vi "UpdateErrorfile.vi"(8 "error in (no error)":errorcluster, 9 "Error file number":u32, 10 "Error file":path, 11 "TCP_serverGUI in":refnum<class "TCP_serverGUI.lvclass">) -> (0 "error out":errorcluster, 3 "TCP_serverGUI out":refnum<class "TCP_serverGUI.lvclass">)   [LabVIEW 2023, in "TCP_serverGUI.lvlib" / "TCP_serverGUI.lvclass"]
uses:
  TCP_serverGUI.lvclass
  TCP_serverGUI.lvclass/TCP_serverGUI.ctl
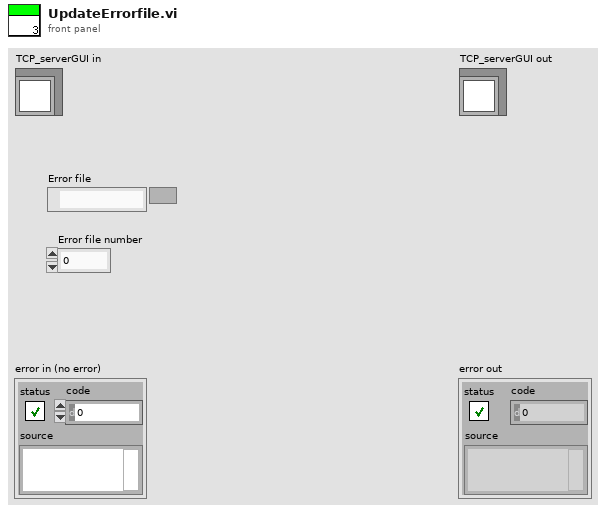
[diagram p1: front panel]
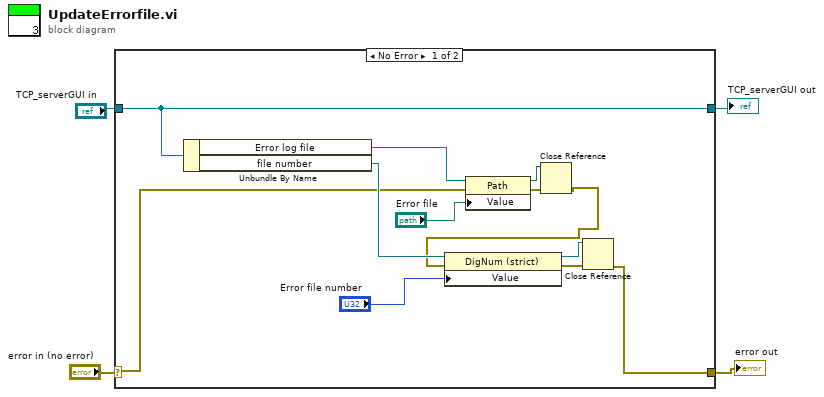
[diagram p0: block diagram]
diagram:
  n1 = case shown="No Error" "error in (no error)" {
    selector: "error in (no error)" -> [w7 w18]
    tunnel: [w5 w18] -> w3
    tunnel: [w16 w17] -> w1
    tunnel: "TCP_serverGUI in" -> [w16 w17]
    frame No Error {
      n2 = Unbundle By Name(w16) -> ("Error log file"=w11:refnum<vi>, "file number"=w10:refnum<vi>)
      n3 = property class="Path"(reference=w11, error in=w7, "Value"="Error file") -> (reference out=w14:refnum<vi>, error out=w15:errorcluster)
      n4 = Close Reference(reference=w14, error in (no error)=w15) -> (error out=w6:errorcluster)
      n5 = property class="DigNum (strict)"(reference=w10, error in=w6, "Value"="Error file number") -> (reference out=w13:refnum<vi>, error out=w12:errorcluster)
      n6 = Close Reference(reference=w13, error in (no error)=w12) -> (error out=w5:errorcluster)
    }
    frame Error {
    }
  }
  "error out" <- w3
  "TCP_serverGUI out" <- w1
